vi "gsp_simulator.vi"() -> ()   [LabVIEW 2015]
panel:
  in  "VISA resource name":refnum<visa-resource-name>="ASRL2::INSTR"
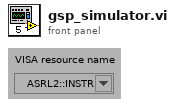
[diagram p1: front panel]
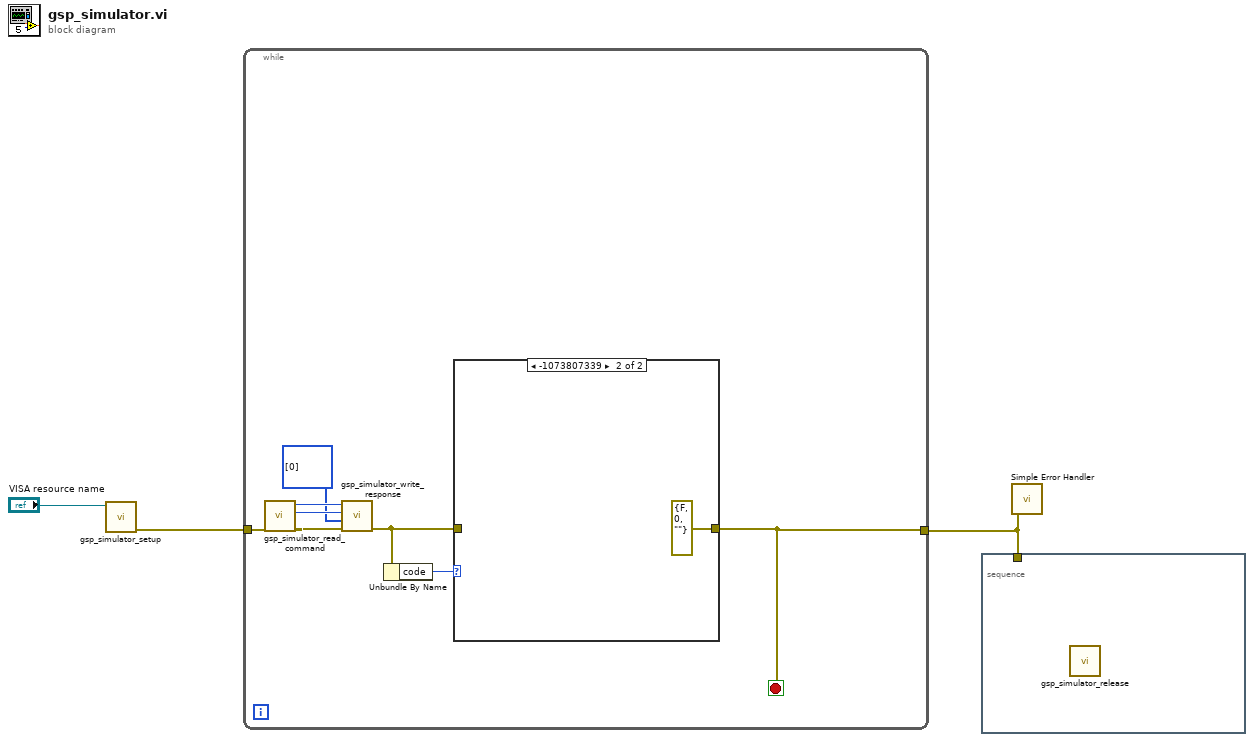
[diagram p0: block diagram]
diagram:
  n1 = call "gsp_simulator_setup.vi"("VISA resource name"="VISA resource name") -> ("error out"=w2:errorcluster)  [unwired: 6 in]
  n2 = while {
    tunnel: w2 -> [w11]
    tunnel: [w5] -> w1
    stop <- w5 stop-if-true
    n3 = call "gsp_simulator_read_command.vi"("error in (no error)"=w11) -> ("error out"=w10:errorcluster, "Motor#"=w8:u8, "Command#"=w9:u16)  [unwired: 3 in, 1 out]
    n4 = call "gsp_simulator_write_response.vi"("error in (no error)"=w10, "Parameters"=i32[] [0], "Motor#"=w8, "Command#"=w9) -> ("error out"=w6:errorcluster)  [unwired: 3 in]
    n5 = Unbundle By Name(w6) -> ("code"=w7:i32)
    n6 = case shown="-1073807339" w7 {
      tunnel: w6 -> [w12 _]
      tunnel: [w12 errorcluster {"status"=FALSE, "code"=0, "source"=""} ("error out")] -> w5
      frame 0, Default {
      }
      frame -1073807339 {
      }
    }
  }
  n7 = stacked-sequence {
    tunnel: w1 -> [_]
    frame #0 {
      n8 = call "gsp_simulator_release.vi"() -> ()  [unwired: 7 in, 1 out]
    }
  }
  n9 = call <vilib>:"Simple Error Handler.vi"("error in (no error)"=w1) -> ()  [unwired: 4 in, 5 out]
